vi "PC_Puck_Position_to_Steps (DONE).vi"(6 "Puck to Step Constants":T2={"Encoder References Positions (steps)"={"X Steps"=100005.0, "Y Steps"=99997.0}, "Encoder References (mm)"={"Encoder References Start Positions (mm)"={"X Steps (Start)"=61.56, "Y Steps (Start)"=7.26}, "Encoder References End Positions (mm)"={"X Steps (End)"=134.65, "Y Steps (End)"=146.25}}, "Encoder References to Dot (steps)"={"Reference X Encoder"=232476.0, "Reference Y Encoder"=229918.0}, "Reference Dot Width (mm)"=14.3}, 7 "Error In":errorcluster, 8 "Puck and Defender Output (pixels)":T3, 9 "Reference Dot Dimentions In (pixels)":cluster{"X":dbl, "Y":dbl, "Width":dbl}) -> (0 "Error Out":errorcluster, 1 "Y Steps to Puck":dbl, 2 "X Steps to Puck":dbl, 3 "Conversions":cluster{dbl, dbl, dbl})   [LabVIEW 2017]
panel:
  in  "Conversions Bundle Names":T1
  out "Y Puck to Dot (steps)":dbl
  out "X Puck to Dot (steps)":dbl
  out "Y Steps/px":dbl
  out "X Steps/px":dbl
  out "Y Steps/mm":dbl
  out "X Steps/mm":dbl
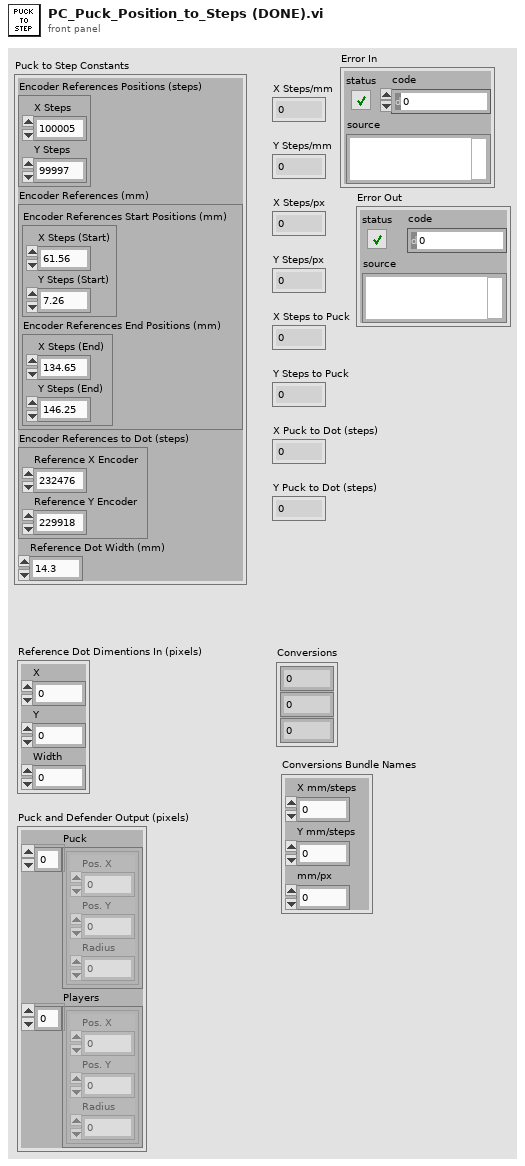
[diagram p1: front panel]
types:
  T1 = cluster{"X mm/steps":dbl, "Y mm/steps":dbl, "mm/px":dbl}
  T2 = cluster{"Encoder References Positions (steps)":cluster{"X Steps":dbl, "Y Steps":dbl}, "Encoder References (mm)":cluster{"Encoder References Start Positions (mm)":cluster{"X Steps (Start)":dbl, "Y Steps (Start)":dbl}, "Encoder References End Positions (mm)":cluster{"X Steps (End)":dbl, "Y Steps (End)":dbl}}, "Encoder References to Dot (steps)":cluster{"Reference X Encoder":dbl, "Reference Y Encoder":dbl}, "Reference Dot Width (mm)":dbl}
  T3 = cluster{"Puck":cluster{"Pos. X":i32, "Pos. Y":i32, "Radius":i32}[], "Players":cluster{"Pos. X":i32, "Pos. Y":i32, "Radius":i32}[]}
  T4 = cluster{"Encoder References Start Positions (mm)":cluster{"X Steps (Start)":dbl, "Y Steps (Start)":dbl}, "Encoder References End Positions (mm)":cluster{"X Steps (End)":dbl, "Y Steps (End)":dbl}}
  T5 = cluster{"Reference X Encoder":dbl, "Reference Y Encoder":dbl}
  T6 = cluster{"Pos. X":i32, "Pos. Y":i32, "Radius":i32}[]
  T7 = cluster{"X Steps (Start)":dbl, "Y Steps (Start)":dbl}
  T8 = cluster{"X Steps (End)":dbl, "Y Steps (End)":dbl}
  T9 = cluster{"Pos. X":i32, "Pos. Y":i32, "Radius":i32}
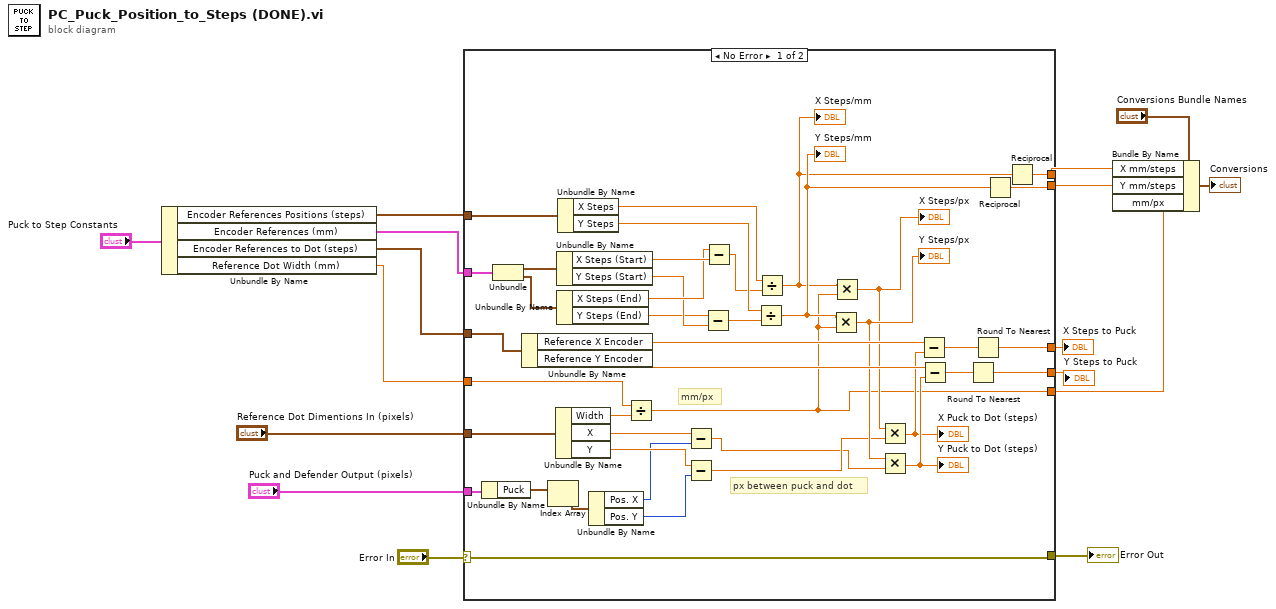
[diagram p0: block diagram]
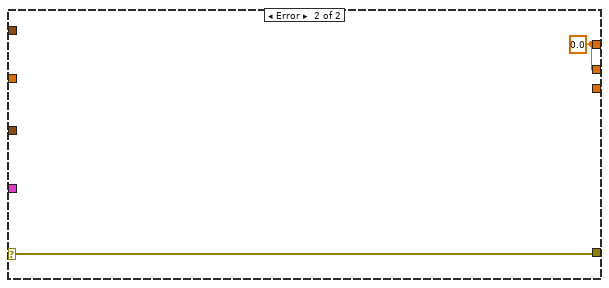
[diagram p2: hidden frame]
diagram:
  n1 = Unbundle By Name("Puck to Step Constants") -> ("Encoder References Positions (steps)"=w9:cluster{"X Steps":dbl, "Y Steps":dbl}, "Encoder References (mm)"=w8:T4, "Encoder References to Dot (steps)"=w7:T5, "Reference Dot Width (mm)"=w6:dbl)
  n2 = case shown="No Error" "Error In" {
    selector: "Error In" -> [w26 w58]
    tunnel: [w22 w59] -> w16
    tunnel: [w23 w59] -> w15
    tunnel: w9 -> [w45 _]
    tunnel: w8 -> [w38 _]
    tunnel: w7 -> [w37 _]
    tunnel: "Puck and Defender Output (pixels)" -> [w32 _]
    tunnel: w6 -> [w29 _]
    tunnel: "Reference Dot Dimentions In (pixels)" -> [w27 _]
    tunnel: [w26 w58] -> w11
    tunnel: [w20 _] -> w5
    tunnel: [w19 _] -> w4
    tunnel: [w18 _] -> w3
    frame No Error {
      # "px between puck and dot"
      # "mm/px"
      n3 = Unbundle By Name(w32) -> ("Puck"=w31:T6)
      n4 = Unbundle(w38) -> ("Encoder References Start Positions (mm)"=w39:T7, "Encoder References End Positions (mm)"=w40:T8)
      n5 = Unbundle By Name(w37) -> ("Reference X Encoder"=w52:dbl, "Reference Y Encoder"=w55:dbl)
      n6 = Index Array(array=w31) -> (element=w30:T9)  [unwired: 1 in]
      n7 = Unbundle By Name(w27) -> ("Width"=w28:dbl, "X"=w33:dbl, "Y"=w35:dbl)
      n8 = Unbundle By Name(w39) -> ("X Steps (Start)"=w44:dbl, "Y Steps (Start)"=w42:dbl)
      n9 = Unbundle By Name(w40) -> ("X Steps (End)"=w43:dbl, "Y Steps (End)"=w41:dbl)
      n10 = Unbundle By Name(w45) -> ("X Steps"=w46:dbl, "Y Steps"=w48:dbl)
      n11 = Unbundle By Name(w30) -> ("Pos. X"=w34:i32, "Pos. Y"=w36:i32)
      n12 = Divide(x=w29, y=w28) -> (x/y=w18:dbl)
      n13 = Subtract(x=w33, y=w34) -> (x-y=w24:dbl)
      n14 = Subtract(x=w35, y=w36) -> (x-y=w25:dbl)
      n15 = Subtract(x=w41, y=w42) -> (x-y=w49:dbl)
      n16 = Subtract(x=w43, y=w44) -> (x-y=w47:dbl)
      n17 = Divide(x=w48, y=w49) -> (x/y=w21:dbl)
      "Y Steps/mm" <- w21
      n18 = Divide(x=w46, y=w47) -> (x/y=w17:dbl)
      "X Steps/mm" <- w17
      n19 = Multiply(x=w21, y=w18) -> (x*y=w51:dbl)
      "Y Steps/px" <- w51
      n20 = Multiply(x=w17, y=w18) -> (x*y=w50:dbl)
      "X Steps/px" <- w50
      n21 = Multiply(x=w50, y=w25) -> (x*y=w53:dbl)
      "X Puck to Dot (steps)" <- w53
      n22 = Multiply(x=w51, y=w24) -> (x*y=w54:dbl)
      "Y Puck to Dot (steps)" <- w54
      n23 = Subtract(x=w52, y=w53) -> (x-y=w56:dbl)
      n24 = Subtract(x=w55, y=w54) -> (x-y=w57:dbl)
      n25 = Round To Nearest(number=w57) -> (nearest integer value=w22:dbl)
      n26 = Round To Nearest(number=w56) -> (nearest integer value=w23:dbl)
      n27 = Reciprocal(x=w21) -> (1/x=w19:dbl)
      n28 = Reciprocal(x=w17) -> (1/x=w20:dbl)
    }
    frame Error {
      w59 = 0.0
    }
  }
  "X Steps to Puck" <- w15
  "Y Steps to Puck" <- w16
  "Error Out" <- w11
  n29 = Bundle By Name(cluster="Conversions Bundle Names", "X mm/steps"=w5, "Y mm/steps"=w4, "mm/px"=w3) -> (→"Conversions":T1)
